vi "Size to Count.vi"(7 "power of 2":i16, 11 "size":u64 format="%08x bytes") -> (3 "count":u64 format="%0d")   [LabVIEW 2017, in "Memory Manager.lvlib" / "Pointer.lvclass"]
doc: "Downshifts <b>size</b> by the specified <b>power of 2</b> to get the count."
uses:
  Pointer.lvclass
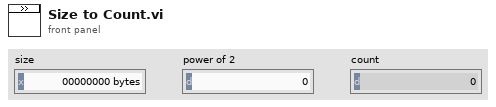
[diagram p1: front panel]
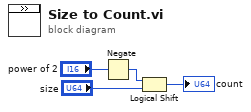
[diagram p0: block diagram]
diagram:
  n1 = Negate(x="power of 2") -> (-x=w1:i16)
  n2 = Logical Shift(y=w1, x="size") -> (x << y=→"count":u64)
